vi "Label Check.vi"(8 "error in (no error)":errorcluster, 9 "Label Black List":string[](array[string]), 10 "Label White List":string[](array[string]), 11 "Label":string) -> (0 "error out":errorcluster, 3 "OK":bool)   [LabVIEW 2021, in "UI-Bus.lvclass"]
uses:
  UI-Bus.lvclass
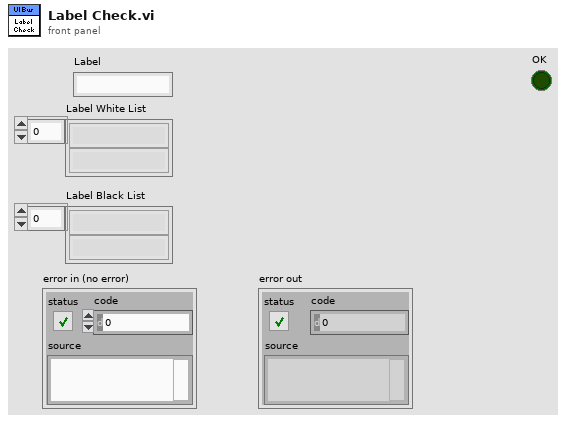
[diagram p1: front panel]
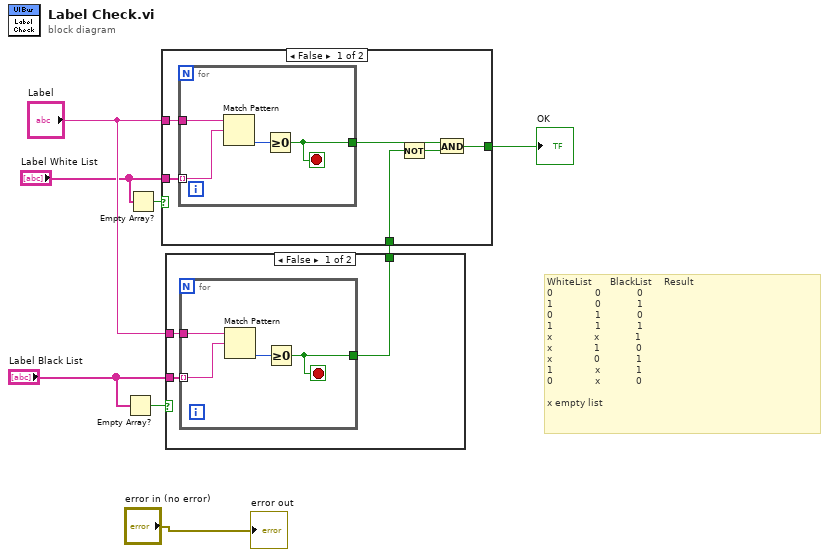
[diagram p0: block diagram]
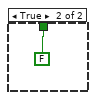
[diagram p2: hidden frame]
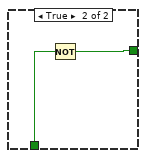
[diagram p3: hidden frame]
diagram:
  # "WhiteList      BlackList    Result\n0              0            0\n1              0            1\n0              1            0\n1              1            1\nx              x            1\nx              1            0\nx              0            1\n1              x            1\n0              x            0\n\nx empty list"
  n1 = Empty Array?(array="Label Black List") -> (empty?=w6:bool)
  n2 = Empty Array?(array="Label White List") -> (empty?=w4:bool)
  n3 = case shown="False" w6 {
    tunnel: "Label Black List" -> [w11 _]
    tunnel: "Label" -> [w10 _]
    tunnel: [w9 FALSE] -> w2
    frame False {
      n4 = for {
        tunnel: w11 -> [w14] mode=indexing
        tunnel: w10 -> [w15]
        tunnel: [w12] -> w9
        stop <- w12 stop-if-true
        n5 = Match Pattern(string=w15, regular expression=w14) -> (offset past match=w13:i32)  [unwired: 1 in, 3 out]
        n6 = Greater Or Equal To 0?(x=w13) -> (x >= 0?=w12:bool)
      }
    }
    frame True {
    }
  }
  n7 = case shown="False" w4 {
    tunnel: "Label White List" -> [w22 _]
    tunnel: "Label" -> [w21 _]
    tunnel: [w19 w27] -> w1
    tunnel: w2 -> [w18 w28]
    frame False {
      n8 = for {
        tunnel: w22 -> [w25] mode=indexing
        tunnel: w21 -> [w26]
        tunnel: [w23] -> w20
        stop <- w23 stop-if-true
        n9 = Match Pattern(string=w26, regular expression=w25) -> (offset past match=w24:i32)  [unwired: 1 in, 3 out]
        n10 = Greater Or Equal To 0?(x=w24) -> (x >= 0?=w23:bool)
      }
      n11 = Not(x=w18) -> (.not. x?=w17:bool)
      n12 = And(x=w20, y=w17) -> (x .and. y?=w19:bool)
    }
    frame True {
      n13 = Not(x=w28) -> (.not. x?=w27:bool)
    }
  }
  "OK" <- w1
  "error out" <- "error in (no error)"
